vi "Set Intensity Graph X Label.vi"(8 "error in (no error)":errorcluster, 10 "X Label":string, 11 "graph_utilities in":refnum<class "graph_utilities.lvclass">) -> (0 "error out":errorcluster, 3 "graph_utilities out":refnum<class "graph_utilities.lvclass">)   [LabVIEW 2016, in "graph_utilities.lvclass"]
doc: "Set the X Label of the Intensity Graph"
uses:
  graph_utilities.lvclass
  graph_utilities.lvclass/graph_utilities.ctl
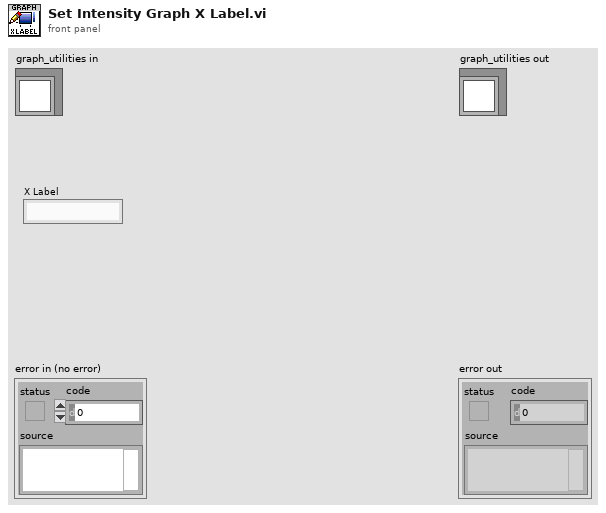
[diagram p1: front panel]
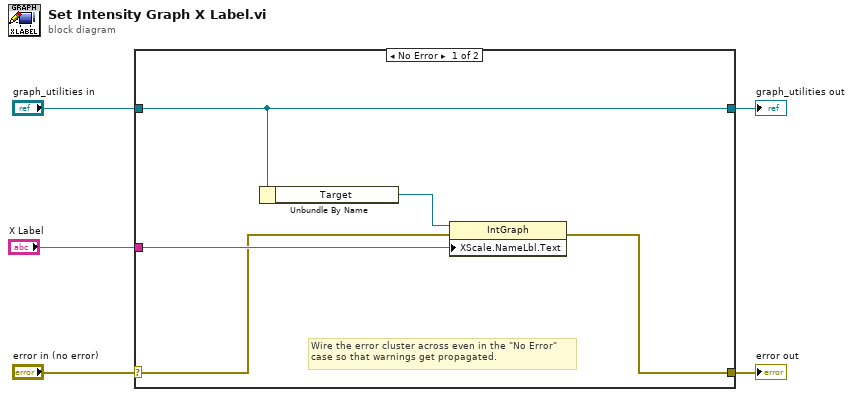
[diagram p0: block diagram]
diagram:
  n1 = case shown="No Error" "error in (no error)" {
    selector: "error in (no error)" -> [w7 w12]
    tunnel: [w6 w12] -> w4
    tunnel: [w9 w11] -> w2
    tunnel: "graph_utilities in" -> [w9 w11]
    tunnel: "X Label" -> [w10 _]
    frame No Error {
      # "Wire the error cluster across even in the \"No Error\"\ncase so that warnings get propagated."
      n2 = Unbundle By Name(w9) -> ("Target"=w8:refnum<vi>)
      n3 = property on="Property Node" class="IntGraph"(reference=w8, error in=w7, "XScale.NameLbl.Text"=w10) -> (error out=w6:errorcluster)  [unwired: 1 out]
    }
    frame Error {
    }
  }
  "error out" <- w4
  "graph_utilities out" <- w2
